vi "PH_Cam_BaseClass.evt call ShowImg.vi"(0 "i ref in":refnum<vi>, 2 "Instance":string, 3 "Start Cam":bool, 5 "error in (no error)":errorcluster) -> (14 "i ref out":refnum<vi>, 19 "error out":errorcluster)   [LabVIEW 2014, in "PH_Cam_BaseClass.lvlib"]
doc: "This VI sends a simple call for ShowImg."
uses:
  CSCore/CSSystem/CoreLib/CoreLib.short 2 byte array.vi
  PH_Cam_BaseClass.lvlib
  CSCore/CSSystem/CoreLib/CoreLib.lvlib
  CSCore/BaseProcess/BaseProcess.lvlib
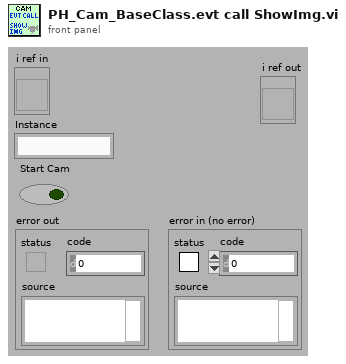
[diagram p1: front panel]
types:
  T1 = typedef "CoreDefs.rawDataType.ctl" = i8[]
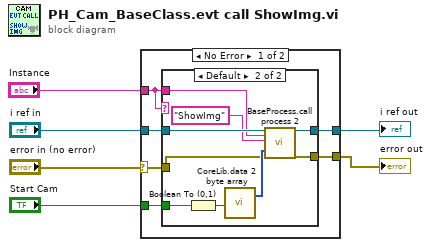
[diagram p0: block diagram]
diagram:
  n1 = case shown="No Error" "error in (no error)" {
    selector: "error in (no error)" -> [w8 w24]
    tunnel: [w12 w25] -> w6
    tunnel: [w11 w24] -> w5
    tunnel: "i ref in" -> [w10 w25]
    tunnel: "Instance" -> [w7 _]
    tunnel: "Start Cam" -> [w9 _]
    frame No Error {
      n2 = case shown="Default" w7 {
        tunnel: [w14 w23] -> w12
        tunnel: [w13 w22] -> w11
        tunnel: w10 -> [w14 w21]
        tunnel: w7 -> [_ w20]
        tunnel: w9 -> [_ w16]
        tunnel: w8 -> [w13 w15]
        frame "N/A" {
        }
        frame Default {
          n3 = Boolean To (0,1)(Boolean=w16) -> (0, 1=w18:i16)
          n4 = call-poly "CoreLib.data 2 byte array.vi"("i16"=w18) -> ("byteArray out"=w17:T1)  [unwired: 18 in]
          n5 = call "BaseProcess.call process 2.vi"("i ref in"=w21, "Object"=w20, "Selector"="ShowImg", "Data"=w17, "error in (no error)"=w15) -> ("i ref out"=w23:refnum<vi>, "error out"=w22:errorcluster)  [unwired: 13 in]
        }
      }
    }
    frame Error {
    }
  }
  "error out" <- w5
  "i ref out" <- w6
